vi "get_puff_stimulus_settings.vi"(1 "Input References Cluster":T1) -> (0 "output values cluster":T2)   [LabVIEW 2015]
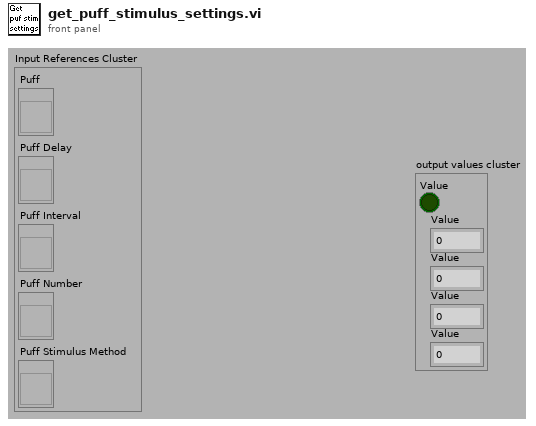
[diagram p1: front panel]
types:
  T1 = cluster{"Puff":refnum<vi>, "Puff Delay":refnum<vi>, "Puff Interval":refnum<vi>, "Puff Number":refnum<vi>, "Puff Stimulus Method":refnum<vi>}
  T2 = cluster{"Value":bool, "Value":dbl, "Value":dbl, "Value":dbl, "Value":u16}
  T3 = cluster{"Value":bool, "Value":dbl, "Value":dbl, "Value":i32, "Value":u16}
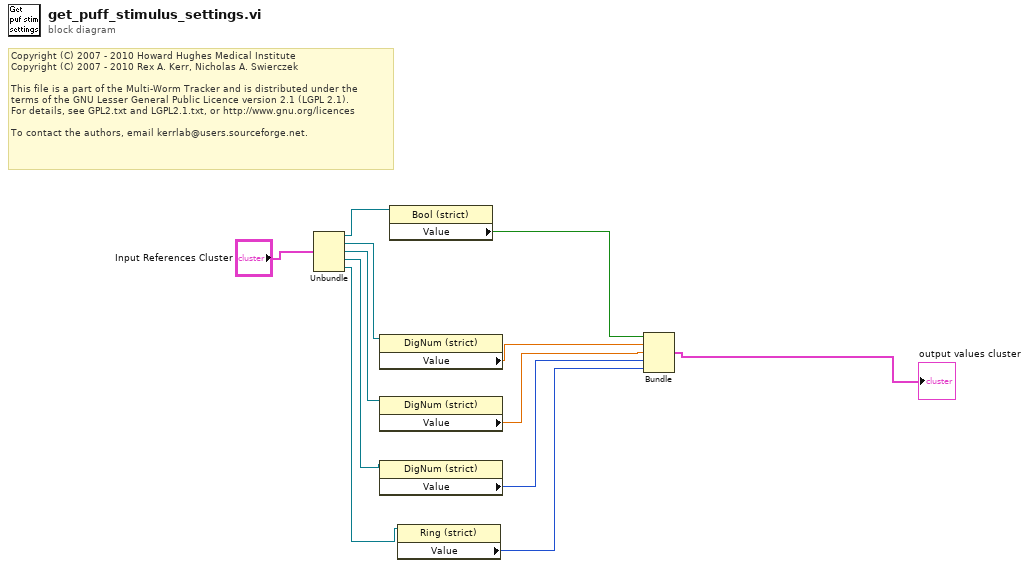
[diagram p0: block diagram]
diagram:
  # "Copyright (C) 2007 - 2010 Howard Hughes Medical Institute\nCopyright (C) 2007 - 2010 Rex A. Kerr, Nicholas A. Swierczek\n \nThis file is a part of the Multi-Worm Tracker and is distributed under the\nterms of the GNU Lesser General Public Licence version 2.1 (LGPL 2.1).\nFor details, see GPL2.txt and LGPL2.1.txt, or http://www.gnu.org/licences\n \nTo contact the authors, email kerrlab@users.sourceforge.net."
  n1 = Unbundle("Input References Cluster") -> ("Puff"=w4:refnum<vi>, "Puff Delay"=w5:refnum<vi>, "Puff Interval"=w6:refnum<vi>, "Puff Number"=w7:refnum<vi>, "Puff Stimulus Method"=w8:refnum<vi>)
  n2 = property class="DigNum (strict)"(reference=w5) -> ("Value"=w12:dbl)  [unwired: 1 in, 2 out]
  n3 = property class="DigNum (strict)"(reference=w6) -> ("Value"=w11:dbl)  [unwired: 1 in, 2 out]
  n4 = property class="DigNum (strict)"(reference=w7) -> ("Value"=w10:i32)  [unwired: 1 in, 2 out]
  n5 = property class="Bool (strict)"(reference=w4) -> ("Value"=w3:bool)  [unwired: 1 in, 2 out]
  n6 = property class="Ring (strict)"(reference=w8) -> ("Value"=w9:u16)  [unwired: 1 in, 2 out]
  n7 = Bundle("Value"=w3, "Value"=w12, "Value"=w11, "Value"=w10, "Value"=w9) -> (→"output values cluster":T3)  [unwired: 1 in]
